vi "Set Units.vi"(8 "error in (no error)":errorcluster, 9 "firmware revision":string(combo), 10 "units (NS)":i32(ring)=1 items=["NS"=1, "DS"=2, "KO"=3, "GO"=4, "JP"=5], 11 "VISA resource name":refnum<visa-resource-name>) -> (0 "error out":errorcluster, 1 "measurement results":T2, 2 "bridge error":T1, 3 "VISA resource name out":refnum<visa-resource-name>)   [LabVIEW 2021, in "Andeen-Hagerling 2700A.lvlib"]
doc: "Selects the units that will be used to report the loss component\nof the measurements.\n\n1 - Nanosiemens (NS)\n2 - Dissipation Factor (DS)\n3 - Series (KO)\n4 - Gigohms (GO)\n5 - Loss Vector (JP)"
uses:
  Andeen-Hagerling 2700A.lvlib
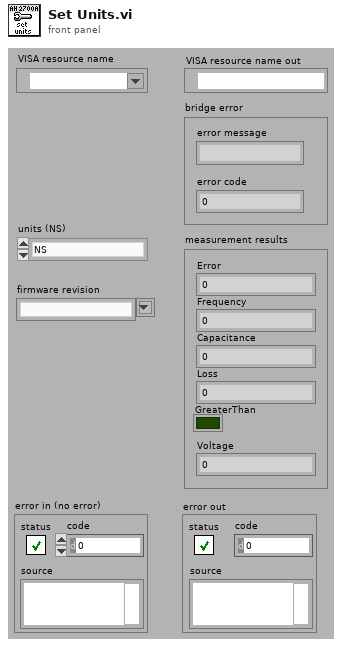
[diagram p1: front panel]
types:
  T1 = cluster{"error message":string, "error code":i32}
  T2 = cluster{"Error":i32, "Frequency":dbl, "Capacitance":dbl, "Loss":dbl, "GreaterThan":bool, "Voltage":dbl}
  T3 = cluster{"error code":i32, "frequency":dbl, "capacitance":dbl, "loss":dbl, "greater than":bool, "voltage":dbl}
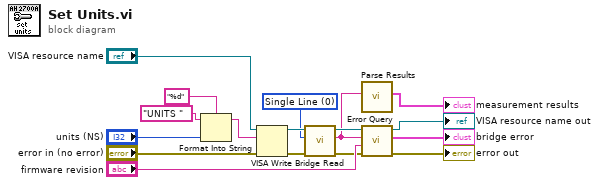
[diagram p0: block diagram]
diagram:
  w1 = u16 0 items=["Single Line", "Multi-Line"] ("Multiline")
  n1 = Format Into String(format string="%d", initial string="UNITS " ("command"), "units (NS)") -> (resulting string=w12:string)  [unwired: 1 in, 1 out]
  n2 = VISA Write(VISA resource name="VISA resource name", write buffer=w12, error in (no error)="error in (no error)") -> (VISA resource name out=w6:refnum<visa-resource-name>, error out=w5:errorcluster)  [unwired: 1 out]
  n3 = call "Bridge Read.vi"("error in (no error)"=w5, "multiline"=w1, "VISA resource name"=w6) -> ("error out"=w2:errorcluster, "read buffer"=w3:string, "VISA resource name out"=w4:refnum<visa-resource-name>)  [unwired: 6 in]
  n4 = call "Parse Results.vi"("measurement line"=w3) -> ("measurement results"=→"measurement results":T3)  [unwired: 9 in]
  n5 = call "Error Query.vi"("error in (no error)"=w2, "firmware revision"="firmware revision", "measurement line"=w3, "VISA resource name"=w4) -> ("error out"=→"error out":errorcluster, "bridge error"=→"bridge error":T1, "VISA resource name out"=→"VISA resource name out":refnum<visa-resource-name>)  [unwired: 5 in]
